vi "Untitled 2.vi"() -> ()   [LabVIEW 2013]
uses:
  <vilib>/express/express arith-compare/Formula/XNode/ExpressFormulaBlockNode.xnode
panel:
  out "obs":string
  in  "Finalizar":bool
  in  "Generar Impar":bool
  out "NumeroImpar":dbl
  in  "GenerarPar":bool
  out "NumeroPar":dbl
  # "Usandon eventos generar un numero par al presionar un generar Par\ny generar un numero impar al presionar un numero Impar."
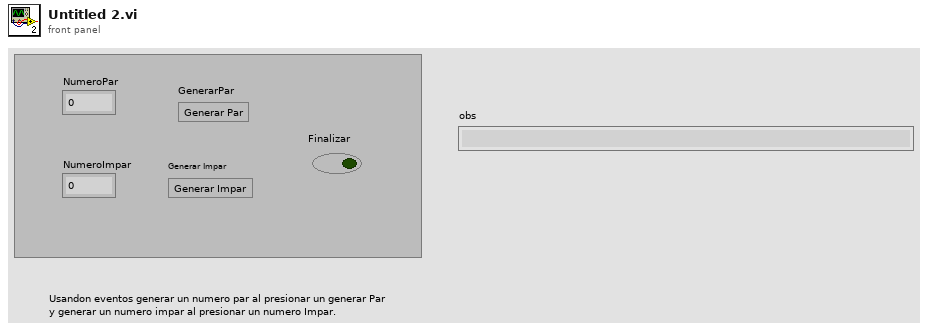
[diagram p1: front panel]
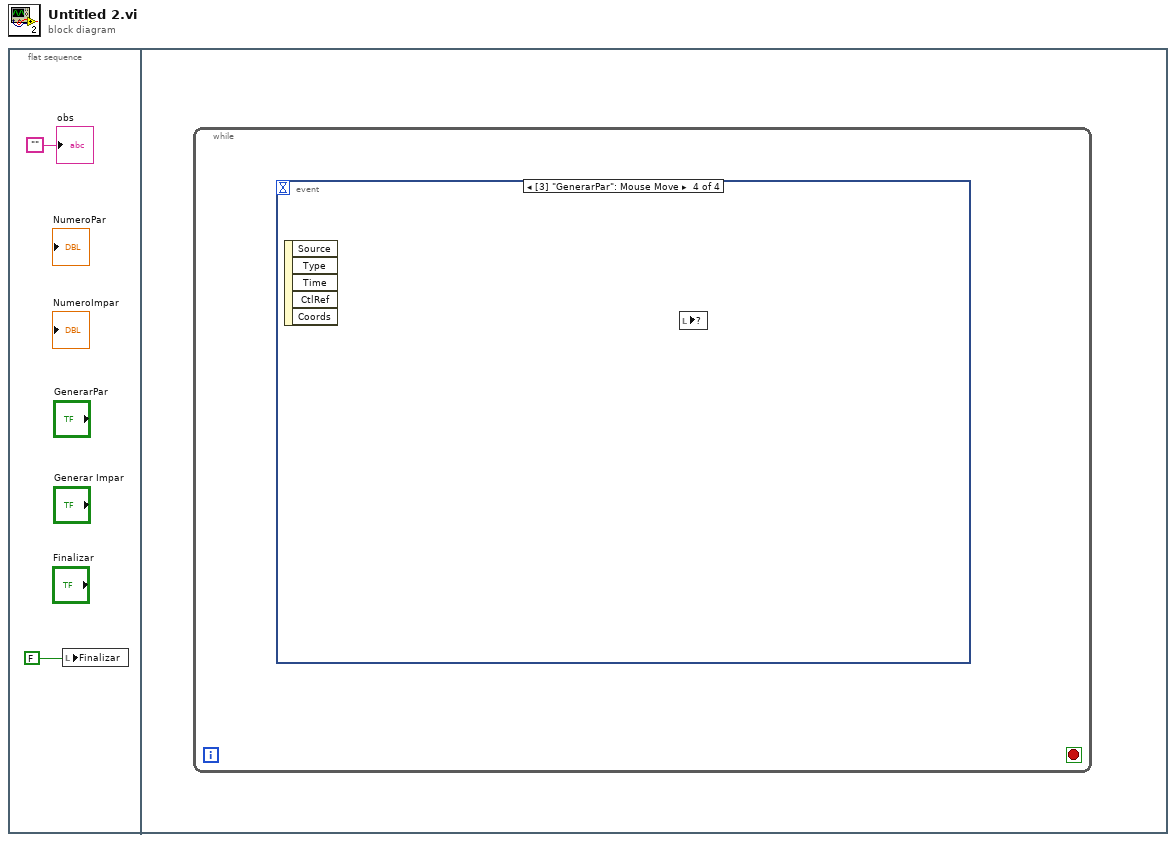
[diagram p0: block diagram]
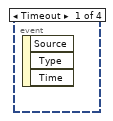
[diagram p2: hidden frame]
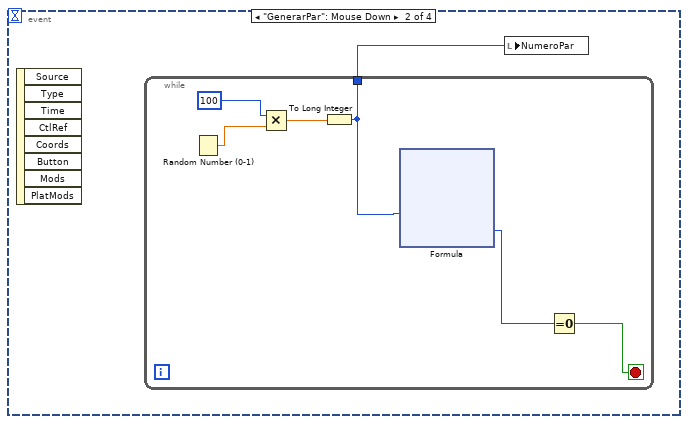
[diagram p3: hidden frame]
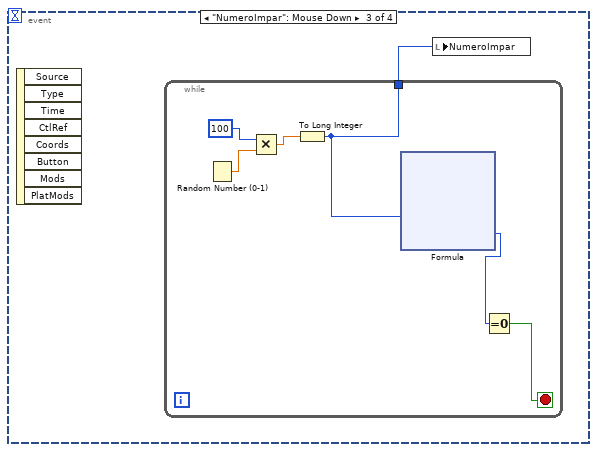
[diagram p4: hidden frame]
diagram:
  n1 = flat-sequence {
    frame #0 {
      n2 = local write "Finalizar"(FALSE) -> ()
      "obs" <- ""
    }
    frame #1 {
      n3 = while {
        stop <- _ stop-if-true
        n4 = event shown="[3] \"GenerarPar\": Mouse Move" {
          selector: _ -> [_ _ _ _]
          dyn-events: _ -> [_ _ _ _]
          timeout: _ -> [_ _ _ _]
          event Timeout {
            n5 = event-data() -> ()  [unwired: 1 in, 3 out]
          }
          event "GenerarPar": Mouse Down {
            n6 = event-data() -> ()  [unwired: 1 in, 8 out]
            n7 = while {
              tunnel: [w4] -> w3
              stop <- w6 stop-if-true
              n8 = Random Number (0-1)() -> (number: 0 to 1=w8:dbl)
              n9 = Multiply(x=100, y=w8) -> (x*y=w7:dbl)
              n10 = To Long Integer(number=w7) -> (32bit integer=w4:i32)
              n11 = xnode "Formula"("X1"=w4) -> ("Result"=w5:i32)  [unwired: 1 in, 1 out]
              n12 = Equal To 0?(x=w5) -> (x = 0?=w6:bool)
            }
            n13 = local write "NumeroPar"(w3) -> ()
          }
          event "NumeroImpar": Mouse Down {
            n14 = event-data() -> ()  [unwired: 1 in, 8 out]
            n15 = while {
              tunnel: [w19] -> w18
              stop <- w20 stop-if-true
              n16 = Random Number (0-1)() -> (number: 0 to 1=w24:dbl)
              n17 = Multiply(x=100, y=w24) -> (x*y=w22:dbl)
              n18 = To Long Integer(number=w22) -> (32bit integer=w19:i32)
              n19 = xnode "Formula"("X1"=w19) -> ("Result"=w21:i32)  [unwired: 1 in, 1 out]
              n20 = Equal To 0?(x=w21) -> (x = 0?=w20:bool)
            }
            n21 = local write "NumeroImpar"(w18) -> ()
          }
          event "GenerarPar": Mouse Move {
            n22 = event-data() -> ()  [unwired: 1 in, 5 out]
            n23 = local read item#-1() -> ()  [unwired: 1 in]
          }
        }
      }
    }
  }
